vi "Driver Remove Summitek Drivers for Spartan 6.0.vi"(8 "error in (no error)":errorcluster) -> (0 "error out":errorcluster)   [LabVIEW 2011]
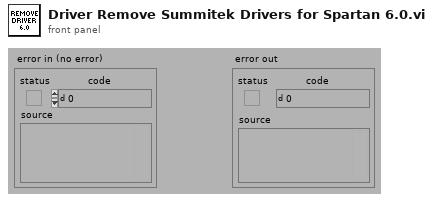
[diagram p1: front panel]
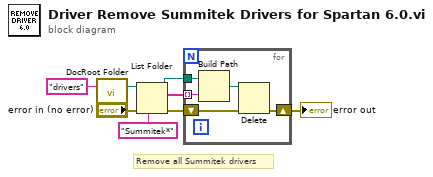
[diagram p0: block diagram]
diagram:
  # "Remove all Summitek drivers"
  n1 = call "DocRoot Folder.vi"("Relative Path (\"\" - Folder)"="drivers" ("Relative Path (\"\" - Folder)")) -> ("DocumentRoot Folder"=w6:path)  [unwired: 2 in]
  n2 = List Folder(path=w6, pattern="Summitek*", error in="error in (no error)") -> (path out=w1:path, filenames=w2:string[], error out=w4:errorcluster)  [unwired: 1 in, 1 out]
  n3 = for {
    shift-right: [w12] -> w3
    shift-left: w4 -> [w13]
    tunnel: w2 -> [w11] mode=indexing
    tunnel: w1 -> [w10]
    n4 = Build Path(base path=w10, name or relative path=w11) -> (appended path=w9:path)
    n5 = Delete(path (use dialog)=w9, error in=w13) -> (error out=w12:errorcluster)  [unwired: 3 in, 2 out]
  }
  "error out" <- w3
